vi "Plot index to active axis.vi"(8 "error in (no error)":errorcluster, 10 "Index":i32, 11 "Plot":refnum<vi>) -> (0 "error out":errorcluster, 2 "Scale reference":refnum<vi>, 3 "Plot":refnum<vi>)   [LabVIEW 2021, in "RocketPlot.lvlib"]
uses:
  RocketPlot.lvlib
  <vilib>/Utility/error.llb/Error Cluster From Error Code.vi
  <vilib>/ErrorRing/Error Ring.xnode
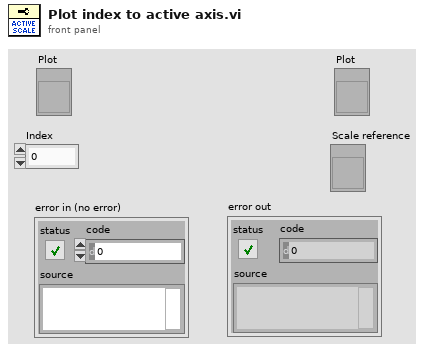
[diagram p1: front panel]
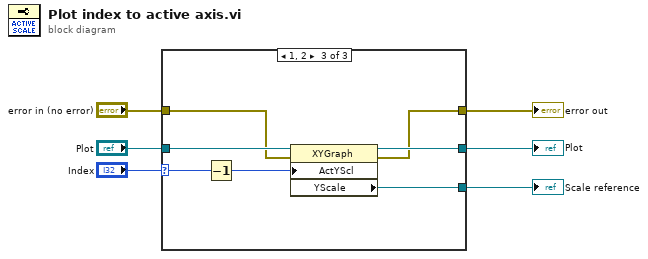
[diagram p0: block diagram]
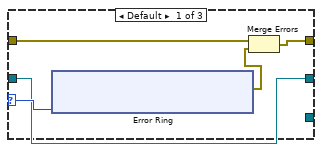
[diagram p2: hidden frame]
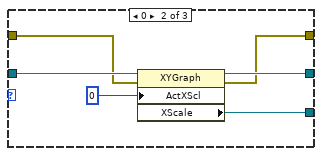
[diagram p3: hidden frame]
diagram:
  n1 = case shown="1, 2" "Index" {
    selector: "Index" -> [w11 _ w26]
    tunnel: "Plot" -> [w7 w24 w31]
    tunnel: [_ w22 w30] -> w5
    tunnel: [w7 w21 w29] -> w4
    tunnel: "error in (no error)" -> [w10 w20 w28]
    tunnel: [w8 w19 w27] -> w2
    frame Default {
      n2 = xnode "Error Ring"("parameter 0"=w11) -> ("error out"=w9:errorcluster)
      n3 = Merge Errors(w10, w9) -> (w8:errorcluster)
    }
    frame 0 {
      n4 = property class="XYGraph"(reference=w24, error in=w20, "ActXScl"=0 ("Active X Scale")) -> (reference out=w21:refnum<vi>, error out=w19:errorcluster, "XScale"=w22:refnum<vi>)
    }
    frame 1, 2 {
      n5 = Decrement(x=w26) -> (x-1=w25:i32)
      n6 = property class="XYGraph"(reference=w31, error in=w28, "ActYScl"=w25) -> (reference out=w29:refnum<vi>, error out=w27:errorcluster, "YScale"=w30:refnum<vi>)
    }
  }
  "error out" <- w2
  "Plot" <- w4
  "Scale reference" <- w5
